vi "Queue Driver.vi"(0 "Enqueue Elements":T2[](array[typedef]), 2 "Name":string, 11 "Error in":errorcluster, 13 "Operations":T1) -> (4 "Dequeued Element":T2, 15 "Error out":errorcluster)   [LabVIEW 2020, in "Data Communication Receiver.lvlib"]
doc: "Queue driver for Receiver to store the states of the receiver."
uses:
  Data Communication Receiver.lvlib
  Typedefs/State and data.ctl
  Typedefs/Queue operations.ctl
panel:
  # "QUEUE DRIVER"
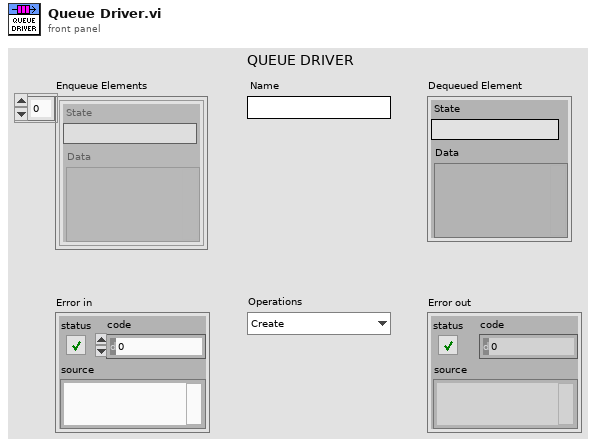
[diagram p1: front panel]
types:
  T1 = typedef "Data Communication Receiver.lvlib/Queue operations.ctl" = enum16{"Create", "Enqueue", "Enstack", "Dequeue", "Flush", "Release"}
  T2 = typedef "Data Communication Receiver.lvlib/State and data.ctl" = cluster{"State":string, "Data":variant}
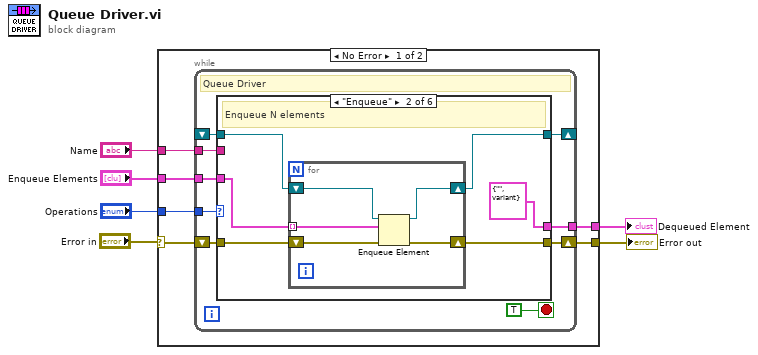
[diagram p0: block diagram]
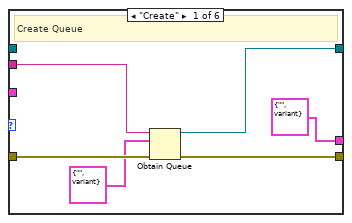
[diagram p2: hidden frame]
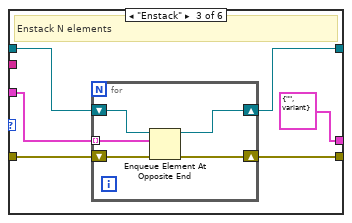
[diagram p3: hidden frame]
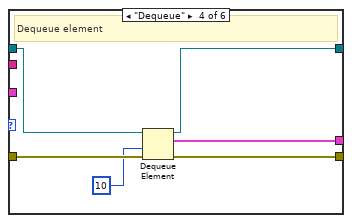
[diagram p4: hidden frame]
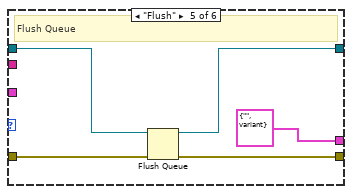
[diagram p5: hidden frame]
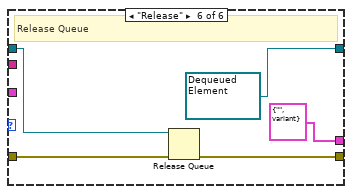
[diagram p6: hidden frame]
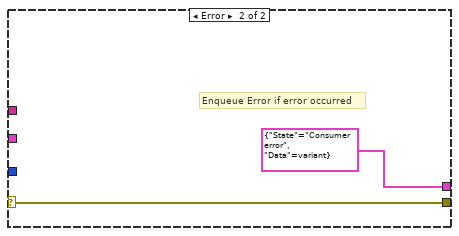
[diagram p7: hidden frame]
diagram:
  n1 = case shown="No Error" "Error in" {
    selector: "Error in" -> [w11 w67]
    tunnel: [w10 w67] -> w5
    tunnel: "Operations" -> [w12 _]
    tunnel: "Name" -> [w9 _]
    tunnel: "Enqueue Elements" -> [w8 _]
    tunnel: [w7 T2 {"State"="Consumer error", "Data"=variant} ("Dequeued Element")] -> w1
    frame No Error {
      n2 = while {
        tunnel: w12 -> [w20]
        tunnel: w9 -> [w17]
        shift-right: [w16] -> _
        shift-left: _ -> [w15]
        tunnel: w8 -> [w14]
        tunnel: [w13] -> w7
        shift-right: [w18] -> w10
        shift-left: w11 -> [w19]
        stop <- TRUE stop-if-true
        # "Queue Driver"
        n3 = case shown="\"Enqueue\"" w20 {
          tunnel: w19 -> [w27 w33 w44 w55 w60 w65]
          tunnel: [w26 w32 w43 w54 w59 w64] -> w18
          tunnel: w17 -> [w25 _ _ _ _ _]
          tunnel: [w23 w31 w42 w51 w57 refnum<queue> refnum ("queue out")] -> w16
          tunnel: w15 -> [_ w30 w41 w52 w56 w63]
          tunnel: w14 -> [_ w29 w40 _ _ _]
          tunnel: [T2 {"State"="", "Data"=variant} ("Dequeued Element") T2 {"State"="", "Data"=variant} ("Dequeued Element") T2 {"State"="", "Data"=variant} ("Dequeued Element") w53 T2 {"State"="", "Data"=variant} ("Dequeued Element") T2 {"State"="", "Data"=variant} ("Dequeued Element")] -> w13
          frame "Create" {
            # "Create Queue"
            n4 = Obtain Queue(name (unnamed)=w25, element data type=T2 {"State"="", "Data"=variant} ("Dequeued Element"), error in (no error)=w27) -> (queue out=w23:refnum<queue>, error out=w26:errorcluster)  [unwired: 2 in, 1 out]
          }
          frame "Enqueue" {
            # "Enqueue N elements"
            n5 = for {
              shift-right: [w37] -> w32
              shift-left: w33 -> [w38]
              tunnel: w29 -> [w34] mode=indexing
              shift-right: [w36] -> w31
              shift-left: w30 -> [w35]
              n6 = Enqueue Element(queue=w35, element=w34, error in (no error)=w38) -> (queue out=w36:refnum<queue>, error out=w37:errorcluster)  [unwired: 1 in, 1 out]
            }
          }
          frame "Enstack" {
            # "Enstack N elements"
            n7 = for {
              shift-right: [w48] -> w43
              shift-left: w44 -> [w49]
              tunnel: w40 -> [w45] mode=indexing
              shift-right: [w47] -> w42
              shift-left: w41 -> [w46]
              n8 = Enqueue Element At Opposite End(queue=w46, element=w45, error in (no error)=w49) -> (queue out=w47:refnum<queue>, error out=w48:errorcluster)  [unwired: 1 in, 1 out]
            }
          }
          frame "Dequeue" {
            # "Dequeue element"
            n9 = Dequeue Element(queue=w52, timeout in ms (-1)=10, error in (no error)=w55) -> (queue out=w51:refnum<queue>, element=w53:T2, error out=w54:errorcluster)  [unwired: 1 out]
          }
          frame "Flush" {
            # "Flush Queue"
            n10 = Flush Queue(queue=w56, error in (no error)=w60) -> (queue out=w57:refnum<queue>, error out=w59:errorcluster)  [unwired: 1 out]
          }
          frame "Release" {
            # "Release Queue"
            n11 = Release Queue(queue=w63, error in (no error)=w65) -> (error out=w64:errorcluster)  [unwired: 1 in, 2 out]
          }
        }
      }
    }
    frame Error {
      # "Enqueue Error if error occurred"
    }
  }
  "Error out" <- w5
  "Dequeued Element" <- w1
